vi "Emergency Send To Specific Target.vi"(6 "Paras In":variant, 8 "error in (no error)":errorcluster, 9 "Mail Strategy In":refnum<class "Mail Strategy.lvclass">, 10 "Message In":refnum<class "Message.lvclass">, 11 "Simple Map Queue Group Messenger in":refnum<class "Simple Map Queue Group Messenger.lvclass">) -> (0 "error out":errorcluster, 3 "Simple Map Queue Group Messenger out":refnum<class "Simple Map Queue Group Messenger.lvclass">)   [LabVIEW 2024, in "Simple Map Queue Group Messenger.lvclass"]
uses:
  Simple Map Queue Group Messenger.lvclass
  Ancestor Class/Message/Message.lvclass
  Ancestor Class/Messenger/Mail Strategy/Mail Strategy.lvclass
  Simple Map Queue Group Messenger.lvclass/Simple Map Queue Group Messenger.ctl
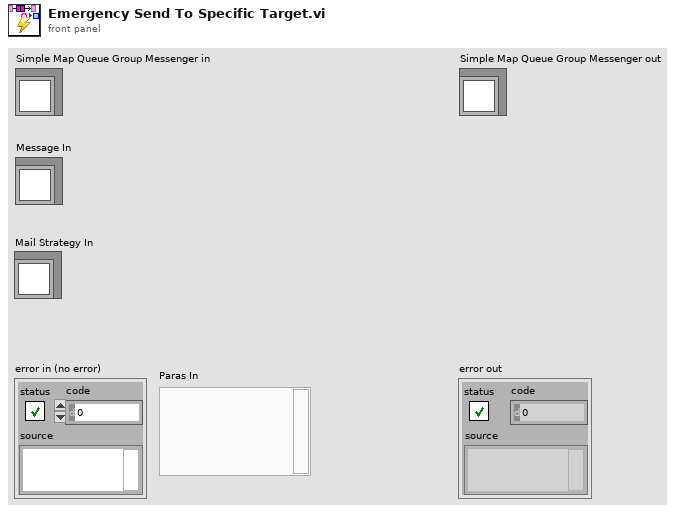
[diagram p1: front panel]
types:
  T1 = typedef "Queue Group Map.ctl" = map{i64, T2[]}
  T2 = typedef "Message Queue.ctl" = refnum<queue>
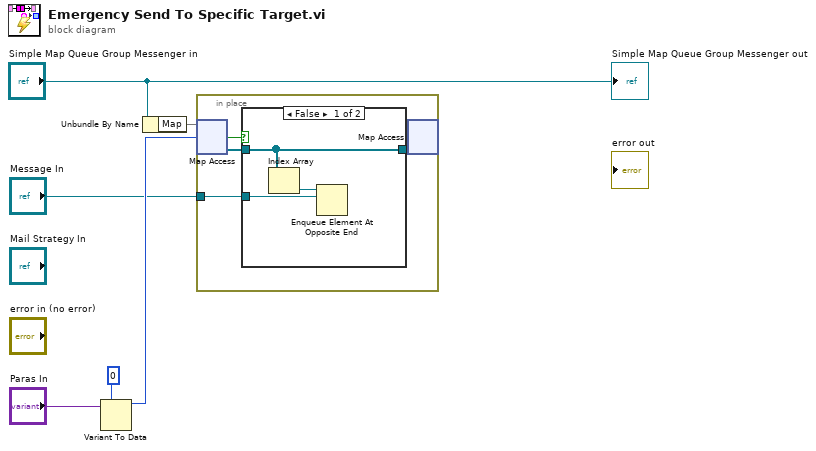
[diagram p0: block diagram]
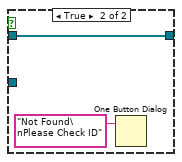
[diagram p2: hidden frame]
diagram:
  n1 = Variant To Data(type=i64 0, Variant="Paras In") -> (data=w2:i64)  [unwired: 1 in, 1 out]
  n2 = Unbundle By Name("Simple Map Queue Group Messenger in") -> ("Map"=w5:T1)
  n3 = in-place {
    in-place-border: "Message In" -> [w7]
    n4 = in-place-map #1(w5, w2) -> (w9:T2[], w10:bool)  [unwired: 1 in]
    n5 = case shown="False" w10 {
      tunnel: w9 -> [w12 w14]
      tunnel: [w12 w14] -> w8
      tunnel: w7 -> [w11 _]
      frame False {
        n6 = Index Array(array=w12) -> (element=w13:T2)  [unwired: 1 in]
        n7 = Enqueue Element At Opposite End(queue=w13, element=w11) -> ()  [unwired: 2 in, 3 out]
      }
      frame True {
        n8 = One Button Dialog(message="Not Found\nPlease Check ID") -> ()  [unwired: 1 in, 1 out]
      }
    }
    n9 = in-place-map #1(w8) -> ()  [unwired: 1 in, 3 out]
  }
  "Simple Map Queue Group Messenger out" <- "Simple Map Queue Group Messenger in"
